vi "Configure Serial Bus (SPI - Source).vi"(0 "VISA resource name":refnum<visa-resource-name>, 1 "MISO Source Channel (0: Channel 1)":i32(ring) items=["Channel 1"=0, "Channel 2"=1, "Channel 3"=2, "Channel 4"=3, "D0"=13, "D1"=14, "D2"=15, "D3"=16, "D4"=17, "D5"=18, "D6"=19, "D7"=20, "D8"=21, "D9"=22, "D10"=23, "D11"=24, "D12"=25, "D13"=26, "D14"=27, "D15"=28, "External"=29], 2 "MOSI Source Channel (1: Channel 2)":i32(ring)=1 items=["Channel 1"=0, "Channel 2"=1, "Channel 3"=2, "Channel 4"=3, "D0"=13, "D1"=14, "D2"=15, "D3"=16, "D4"=17, "D5"=18, "D6"=19, "D7"=20, "D8"=21, "D9"=22, "D10"=23, "D11"=24, "D12"=25, "D13"=26, "D14"=27, "D15"=28, "External"=29], 3 "Clock Source Channel (2: Channel 3)":i32(ring)=2 items=["Channel 1"=0, "Channel 2"=1, "Channel 3"=2, "Channel 4"=3, "D0"=13, "D1"=14, "D2"=15, "D3"=16, "D4"=17, "D5"=18, "D6"=19, "D7"=20, "D8"=21, "D9"=22, "D10"=23, "D11"=24, "D12"=25, "D13"=26, "D14"=27, "D15"=28, "External"=29], 5 "Serial Bus Name (1: Serial Bus 1)":i32(ring)=1 items=["Serial Bus 1"=1, "Serial Bus 2"=2], 7 "Enable Frame Source (F: Disable)":bool, 9 "Frame Source Channel (3: Channel 4)":i32(ring)=3 items=["Channel 1"=0, "Channel 2"=1, "Channel 3"=2, "Channel 4"=3, "D0"=13, "D1"=14, "D2"=15, "D3"=16, "D4"=17, "D5"=18, "D6"=19, "D7"=20, "D8"=21, "D9"=22, "D10"=23, "D11"=24, "D12"=25, "D13"=26, "D14"=27, "D15"=28, "External"=29], 11 "error in (no error)":errorcluster) -> (4 "VISA resource name out":refnum<visa-resource-name>, 15 "error out":errorcluster)   [LabVIEW 2023, in "Keysight-DSQx3014T.lvlib"]
doc: "Configures the source settings of SPI bus."
uses:
  Keysight-DSQx3014T.lvlib
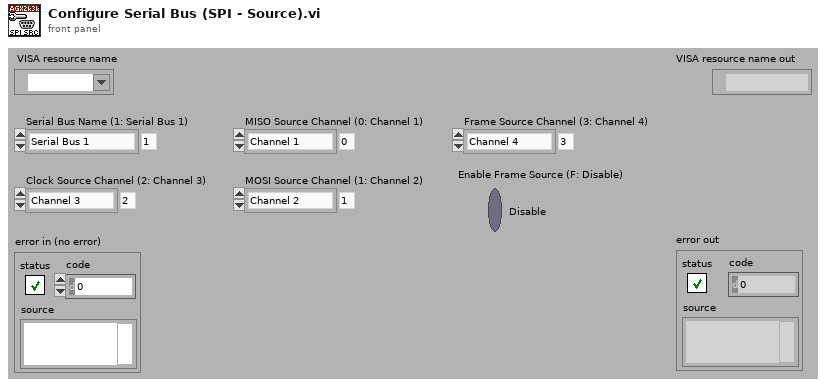
[diagram p1: front panel]
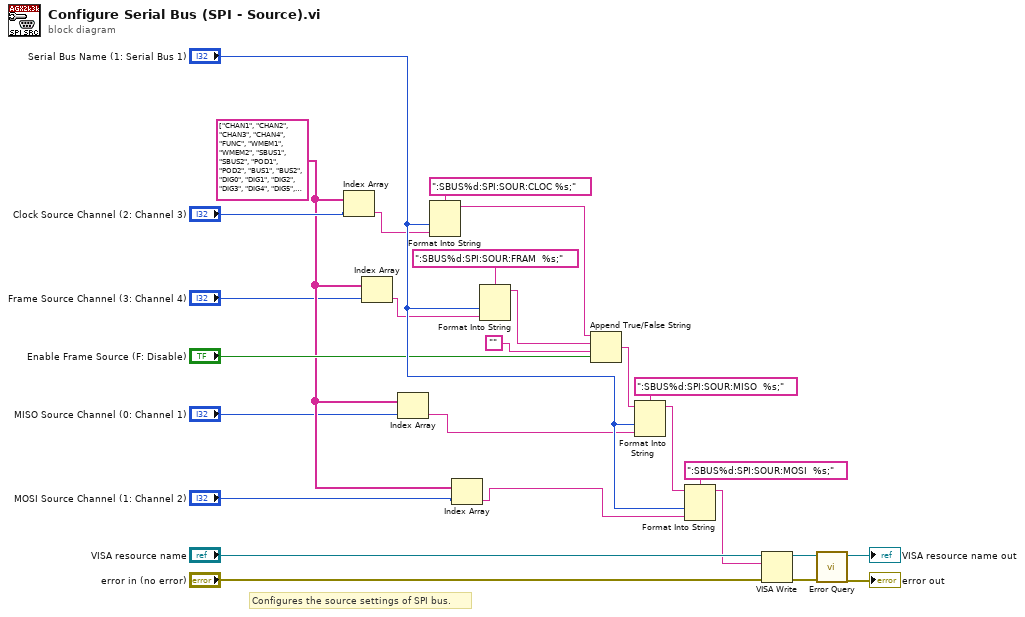
[diagram p0: block diagram]
diagram:
  w5 = string[] ["CHAN1", "CHAN2", "CHAN3", "CHAN4", "FUNC", "WMEM1", "WMEM2", "SBUS1", "SBUS2", "POD1", "POD2", "BUS1", "BUS2", "DIG0", "DIG1", "DIG2", "DIG3", "DIG4", "DIG5", "DIG6", "DIG7", "DIG8", "DIG9", "DIG10", "DIG11", "DIG12", "DIG13", "DIG14", "DIG15", "EXT", "LINE", "WGEN"]
  # "Configures the source settings of SPI bus."
  n1 = Index Array(array=w5, index="Clock Source Channel (2: Channel 3)") -> (element=w9:string)
  n2 = Index Array(array=w5, index="Frame Source Channel (3: Channel 4)") -> (element=w1:string)
  n3 = Index Array(array=w5, index="MISO Source Channel (0: Channel 1)") -> (element=w4:string)
  n4 = Format Into String(format string=":SBUS%d:SPI:SOUR:CLOC %s;", "Serial Bus Name (1: Serial Bus 1)", w9) -> (resulting string=w15:string)  [unwired: 2 in, 1 out]
  n5 = Index Array(array=w5, index="MOSI Source Channel (1: Channel 2)") -> (element=w7:string)
  n6 = Format Into String(format string=":SBUS%d:SPI:SOUR:FRAM  %s;", "Serial Bus Name (1: Serial Bus 1)", w1) -> (resulting string=w14:string)  [unwired: 2 in, 1 out]
  n7 = Append True/False String(1:"Enable Frame Source (F: Disable)", 2:"", 3:w14, 4:w15) -> (0:w12:string)
  n8 = Format Into String(format string=":SBUS%d:SPI:SOUR:MISO  %s;", initial string=w12, "Serial Bus Name (1: Serial Bus 1)", w4) -> (resulting string=w23:string)  [unwired: 1 in, 1 out]
  n9 = Format Into String(format string=":SBUS%d:SPI:SOUR:MOSI  %s;", initial string=w23, "Serial Bus Name (1: Serial Bus 1)", w7) -> (resulting string=w11:string)  [unwired: 1 in, 1 out]
  n10 = VISA Write(VISA resource name="VISA resource name", write buffer=w11, error in (no error)="error in (no error)") -> (VISA resource name out=w19:refnum<visa-resource-name>, error out=w18:errorcluster)  [unwired: 1 out]
  n11 = call "Error Query.vi"("error in (no error)"=w18, "VISA resource name"=w19) -> ("error out"=→"error out":errorcluster, "VISA resource name out"=→"VISA resource name out":refnum<visa-resource-name>)  [unwired: 8 out]
